vi "Configure AWGN ARB.vi"(6 "AWGN Noise Seed (0: Fixed)":u16(ring) items=["Fixed", "Random"], 7 "Enable AWGN ARB (T:Enable)":bool=TRUE, 8 "error in (no error)":errorcluster, 9 "Waveform Length (1: 524288)":u16(ring)=1 items=["1048576", "524288", "262144", "131072", "65536", "32768", "16384"], 10 "AWGN Bandwidth (1 MHz)":dbl=1000000.0, 11 "VISA resource name":refnum<visa-resource-name>) -> (0 "error out":errorcluster, 3 "VISA resource name out":refnum<visa-resource-name>)   [LabVIEW 2018, in "Agilent PSG MXG Series.lvlib"]
doc: "Configures the state, bandwidth, length and noise seed of AWGN (additive white Gaussian noise) ARB.\n\n<B>Notes:</B>\n(1) This VI is valid only in E8257D, E8267D that install <B>Option 403</B> (Calibrated noise, AWGN)."
uses:
  Agilent PSG MXG Series.lvlib
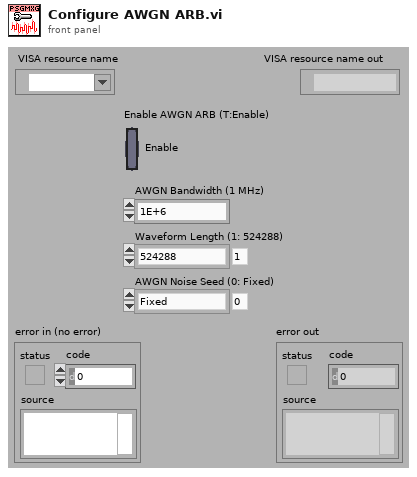
[diagram p1: front panel]
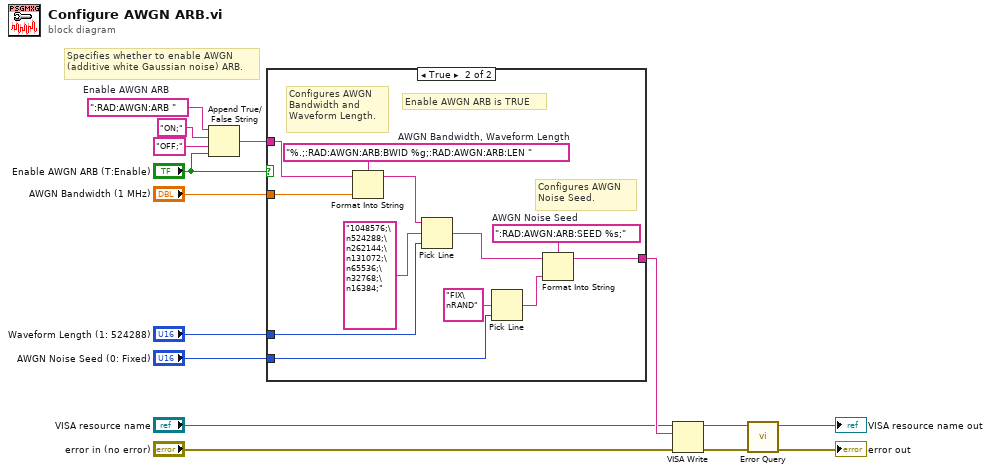
[diagram p0: block diagram]
diagram:
  w15 = ":RAD:AWGN:ARB "  # Enable AWGN ARB
  # "Specifies whether to enable AWGN\n(additive white Gaussian noise) ARB."
  n1 = Append True/False String(1:"Enable AWGN ARB (T:Enable)", 2:"OFF;" ("false string"), 3:"ON;" ("true string"), 4:w15) -> (0:w12:string)
  n2 = case shown="True" "Enable AWGN ARB (T:Enable)" {
    tunnel: w12 -> [w16 w28]
    tunnel: "AWGN Bandwidth (1 MHz)" -> [_ w26]
    tunnel: "Waveform Length (1: 524288)" -> [_ w23]
    tunnel: "AWGN Noise Seed (0: Fixed)" -> [_ w18]
    tunnel: [w16 w17] -> w8
    frame False {
      # "Enable AWGN ARB is FALSE"
    }
    frame True {
      w21 = ":RAD:AWGN:ARB:SEED %s;"  # AWGN Noise Seed
      w27 = "%.;:RAD:AWGN:ARB:BWID %g;:RAD:AWGN:ARB:LEN "  # AWGN Bandwidth, Waveform Length
      # "Enable AWGN ARB is TRUE"
      # "Configures AWGN\nNoise Seed."
      # "Configures AWGN\nBandwidth and\nWaveform Length."
      n3 = Format Into String(format string=w27, initial string=w28, w26) -> (resulting string=w25:string)  [unwired: 1 in, 1 out]
      n4 = Pick Line(string ("")=w25, multi-line string="1048576;\n524288;\n262144;\n131072;\n65536;\n32768;\n16384;", line index=w23) -> (output string=w22:string)
      n5 = Pick Line(multi-line string="FIX\nRAND", line index=w18) -> (output string=w20:string)  [unwired: 1 out]
      n6 = Format Into String(format string=w21, initial string=w22, w20) -> (resulting string=w17:string)  [unwired: 1 in, 1 out]
    }
  }
  n7 = VISA Write(VISA resource name="VISA resource name", write buffer=w8, error in (no error)="error in (no error)") -> (VISA resource name out=w7:refnum<visa-resource-name>, error out=w6:errorcluster)  [unwired: 1 out]
  n8 = call "Error Query.vi"("error in (no error)"=w6, "VISA resource name"=w7) -> ("error out"=→"error out":errorcluster, "VISA resource name out"=→"VISA resource name out":refnum<visa-resource-name>)  [unwired: 8 out]
